vi "Robot Global Data.vi"() -> ()   [LabVIEW 2016]
doc: "This global VI can contain as many global variables as you need. Place a control on the panel, give it a good name. To read or write to it from a VI, drag the icon to the diagram of that VI. You can also drag from the project. Click on the node to change which global you access. You shouldn't have multiple locations writing to a global or it will cause a race-condition."
uses:
  <vilib>/Rock Robotics/WPI/Camera/WPI_CameraImageSize.ctl
  <vilib>/Rock Robotics/WPI/DriverStation/WPI_DriverStationRobotMode2.ctl
  Controls/Auto Selector.ctl
panel:
  in  "Gear in?":bool
  out "Intake speed":dbl
  in  "Targets Found":dbl
  in  "Auto Vision":bool
  in  "Auto Mode":T1
  out "Auto Turret":dbl
  in  "Auto - Prepare Airship":bool
  in  "Auto - Prepare Boiler":bool
  in  "Auto - shoot":bool
  in  "Auto - Gear Manipulator":bool
  out "Auto Distance":dbl
  out "Yaw":dbl
  in  "Reset Grayhill":bool
  out "Auto Right Drive":dbl
  out "Auto Left drive":dbl
  in  "Auto aim locked?":bool
  in  "Top Ready?":bool
  in  "Bot Ready?":bool
  out "Liquidificador %":dbl
  out "Joy 0 Buttons":T2
  out "Gambiarra n1":dbl
  out "Alinhador Setpoint":dbl
  out "Encoder Alinhador":dbl
  out "InitTimer":dbl
  in  "AutoGear":bool
  out "Eixos Xbox":T3
  out "Left Rumble":dbl
  out "Right Rumble":dbl
  out "POV Xbox":T4
  in  "Hood":bool
  out "Indexer %":dbl
  out "Turret Setpoint":dbl
  out "Bot Setpoint":dbl
  out "Top Setpoint":dbl
  out "Buttons Xbox":T2
  out "Eixos Joystick 1":T3
  out "Eixos Joystick 0":T3
  in  "Turret Reset":bool
  out "Turret Angle":dbl
  out "Bot RPM":dbl
  out "Top RPM":dbl
  out "Angle Offset":dbl
  in  "Robot Mode":T5
  in  "image size":T6=enum."320x240"
  in  "Enable Vision":bool
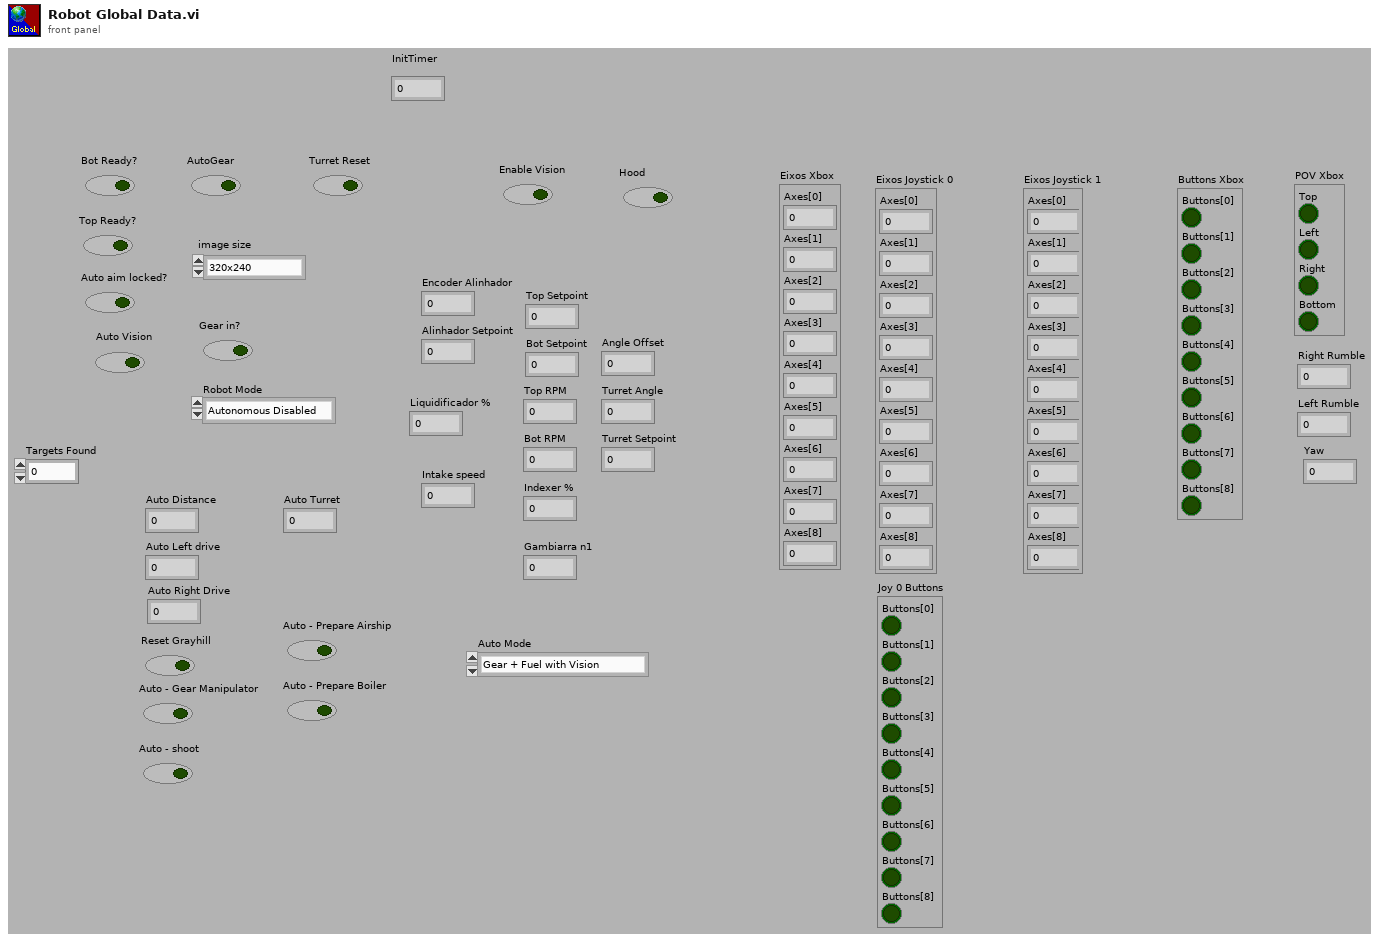
[diagram p1: front panel]
types:
  T1 = typedef "Auto Selector.ctl" = enum16{"Gear + Fuel with Vision", "Gear + Fuel no Vision", "Middle Gear", "Nothing"}
  T2 = cluster{"Buttons[0]":bool, "Buttons[1]":bool, "Buttons[2]":bool, "Buttons[3]":bool, "Buttons[4]":bool, "Buttons[5]":bool, "Buttons[6]":bool, "Buttons[7]":bool, "Buttons[8]":bool}
  T3 = cluster{"Axes[0]":dbl, "Axes[1]":dbl, "Axes[2]":dbl, "Axes[3]":dbl, "Axes[4]":dbl, "Axes[5]":dbl, "Axes[6]":dbl, "Axes[7]":dbl, "Axes[8]":dbl}
  T4 = cluster{"Top":bool, "Left":bool, "Right":bool, "Bottom":bool}
  T5 = typedef "WPI_DriverStationRobotMode2.ctl" = enum16{"Autonomous Disabled", "Autonomous Enabled", "Teleop Disabled", "Teleop Enabled", "Disconnected", "Finish", "Test Disabled", "Test Enabled", "Emergency Stopped"}
  T6 = typedef "WPI_CameraImageSize.ctl" = enum16{"640x480", "320x240", "160x120", "Custom"}
diagram:
